vi "DriveSpeedDemandRateLimit.vi"(8 "PassThrough":dbl=-1.0 format="%33.4f", 11 "inChassisSpeedDemand":T1 {"vOmega" format="%10.3f"; "vY" format="%10.3f"; "vX" format="%10.3f"}) -> (3 "outChassisSpeedDemand":T1 {"vOmega" format="%10.3f"; "vY" format="%10.3f"; "vX" format="%10.3f"})   [LabVIEW 2023]
doc: "Get speed demand variable for drive"
uses:
  <vilib>/Rock Robotics/WPI/ThirdParty/JAS_Junk/TrajLib/TypeDef/CHASSIS_SPEEDS.ctl
  <vilib>/Rock Robotics/WPI/ThirdParty/JAS_Junk/TrajLib/SlewRateLimiter_New.vi
  <vilib>/Rock Robotics/WPI/ThirdParty/JAS_Junk/TrajLib/SlewRateLimiter_Reset.vi
  <vilib>/Rock Robotics/WPI/ThirdParty/JAS_Junk/TrajLib/SlewRateLimiter_Calculate.vi
  <vilib>/Rock Robotics/WPI/ThirdParty/JAS_Junk/TrajLib/SlewRateLimiter_SetRate.vi
  <vilib>/Rock Robotics/WPI/ThirdParty/JAS_Junk/TrajLib/VI/Util_GetTime_U32.vi
  DriveGlobal.vi
  <vilib>/Rock Robotics/WPI/ThirdParty/JAS_Junk/TrajLib/VI/Util_GetTime_U64.vi
  <vilib>/Rock Robotics/WPI/ThirdParty/JAS_Junk/TrajLib/Trajectory_Library.lvlib
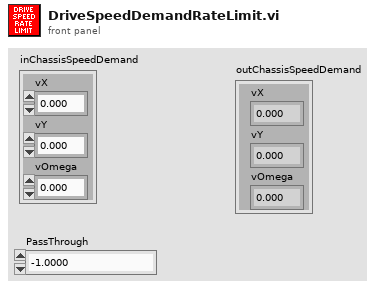
[diagram p1: front panel]
types:
  T1 = typedef "Trajectory_Library.lvlib/CHASSIS_SPEEDS.ctl" = cluster{"vX":dbl, "vY":dbl, "vOmega":dbl}
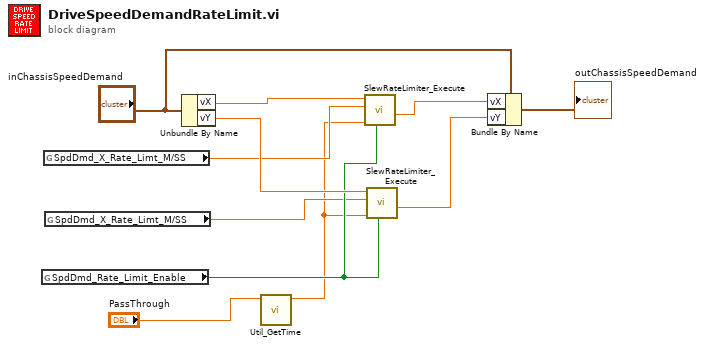
[diagram p0: block diagram]
diagram:
  n1 = global read "DriveGlobal.vi" "SpdDmd_Rate_Limit_Enable"() -> (w5:bool)
  n2 = global read "DriveGlobal.vi" "SpdDmd_X_Rate_Limt_M/SS"() -> (w4:dbl)
  n3 = global read "DriveGlobal.vi" "SpdDmd_X_Rate_Limt_M/SS"() -> (w3:dbl)
  n4 = Unbundle By Name("inChassisSpeedDemand") -> ("vX"=w9:dbl, "vY"=w7:dbl)
  n5 = call <vilib>:"Util_GetTime.vi"("Pass_Through_Time"="PassThrough") -> ("FPGA_Time_Seconds"=w1:dbl)  [unwired: 8 in, 2 out]
  n6 = call <vilib>:"SlewRateLimiter_Execute.vi"("Enable"=w5, "Time"=w1, "PositiveRate"=w4, "Input"=w9) -> ("Output"=w8:dbl)  [unwired: 6 in, 1 out]
  n7 = call <vilib>:"SlewRateLimiter_Execute.vi"("Enable"=w5, "Time"=w1, "PositiveRate"=w3, "Input"=w7) -> ("Output"=w6:dbl)  [unwired: 6 in, 1 out]
  n8 = Bundle By Name(cluster="inChassisSpeedDemand", "vX"=w8, "vY"=w6) -> (→"outChassisSpeedDemand":T1)
